vi "LogCurrentVIName.vi"(8 "error in (no error)":errorcluster, 10 "AdditionalInfo":string) -> (0 "error out":errorcluster)   [LabVIEW 2014, in "GCMLog.lvclass"]
uses:
  GCMLog.lvclass
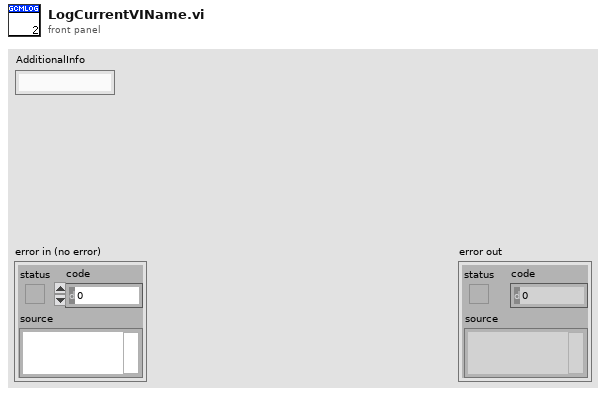
[diagram p1: front panel]
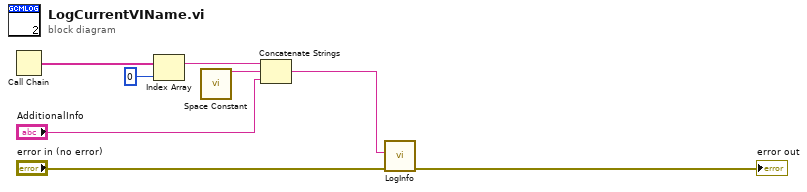
[diagram p0: block diagram]
diagram:
  n1 = Call Chain() -> (call chain=w6:string[])
  n2 = Index Array(array=w6, index=0) -> (element=w5:string)
  n3 = call <vilib>:"Space Constant.vi"() -> ("String"=w1:string)
  n4 = Concatenate Strings(w5, w1, "AdditionalInfo") -> (w3:string)
  n5 = call "LogInfo.vi"("error in (no error)"="error in (no error)", "Info"=w3) -> ("error out"=→"error out":errorcluster)  [unwired: 9 in]
